vi "Stop.vi"(8 "error in (no error)":errorcluster, 9 "timeout in ms (-1)":i32=-1, 11 "Test Runner In":refnum<class "Test Runner.lvclass">) -> (0 "error out":errorcluster, 1 "timed out?":bool, 3 "Test Runner Out":refnum<class "Test Runner.lvclass">)   [LabVIEW 2020, in "Test Runner.lvclass"]
doc: "Sends a stop message to the process, which must perform a safe shut down. This VI waits for the process to call the Finish method or times out if the configured time out expires."
uses:
  Test Runner.lvclass
  Application Framework/Process Classes/Process/Process.lvclass
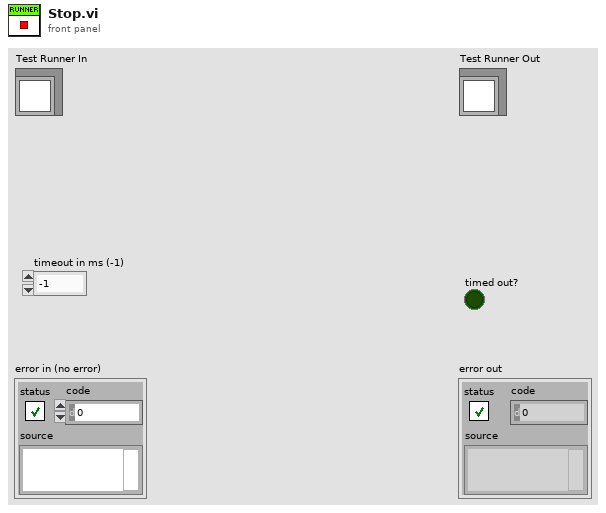
[diagram p1: front panel]
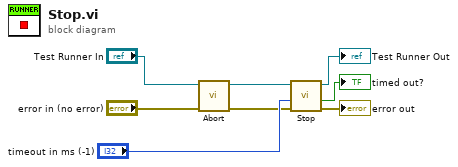
[diagram p0: block diagram]
diagram:
  n1 = call "Abort.vi"("error in (no error)"="error in (no error)", "Test Runner In"="Test Runner In") -> ("error out"=w3:errorcluster, "Test Runner Out"=w1:refnum<class "Test Runner.lvclass">)  [unwired: 8 in]
  n2 = call-parent "Stop.vi"("error in (no error)"=w3, "timeout in ms (-1)"="timeout in ms (-1)", "Process In"=w1) -> ("error out"=→"error out":errorcluster, "timed out?"=→"timed out?":bool, "Process Out"=→"Test Runner Out":refnum<class "Test Runner.lvclass">)  [unwired: 6 in]
